vi "Init.vi"(0 "object in":refnum<class "Scripting.lvclass">, 1 "FindAnyOfTheseClassTypes":string[](array[string]), 2 "StopWhenAnyOfTheseClassTypesAreReached":string[](array[string]), 3 "KeepObjectsOpen(True)":bool=TRUE, 4 "DeleteWires(False)":bool, 5 "error in (no error)":errorcluster) -> (14 "object out":refnum<class "Scripting.lvclass">, 19 "error out":errorcluster)   [LabVIEW 2020, in "Scripting.lvclass"]
uses:
  <resource>/Framework/Providers/Open_GDS/ClassProviders/Common/ScriptingFunctions/Scripting.lvclass
  <resource>/Framework/Providers/Open_GDS/ClassProviders/Common/ScriptingFunctions/Scripting.lvclass/Scripting.ctl
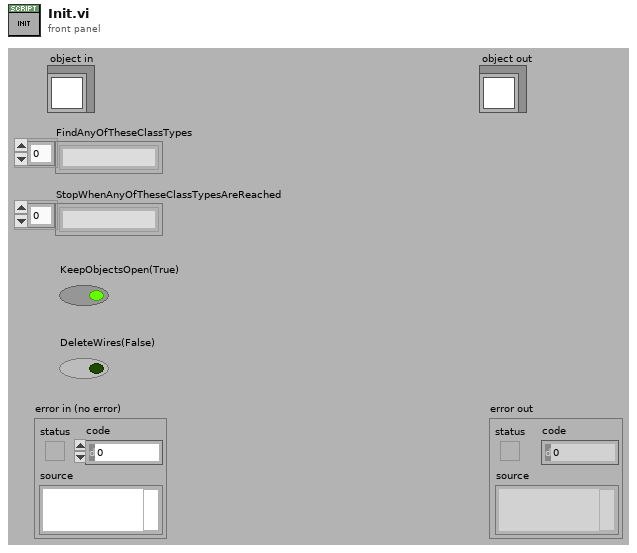
[diagram p1: front panel]
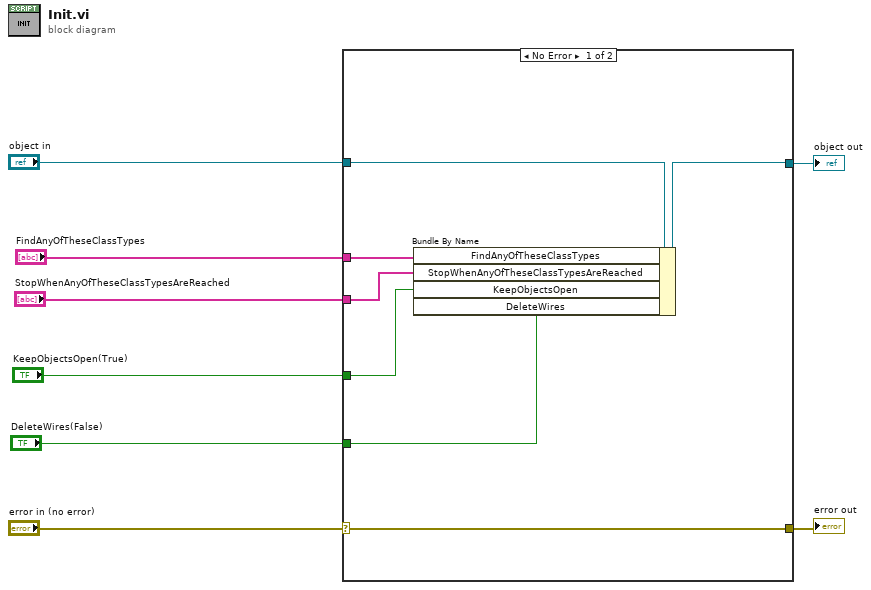
[diagram p0: block diagram]
diagram:
  n1 = case shown="No Error" "error in (no error)" {
    selector: "error in (no error)" -> [w15 w17]
    tunnel: [w15 w17] -> w7
    tunnel: [w13 w16] -> w5
    tunnel: "object in" -> [w14 w16]
    tunnel: "FindAnyOfTheseClassTypes" -> [w12 _]
    tunnel: "StopWhenAnyOfTheseClassTypesAreReached" -> [w11 _]
    tunnel: "KeepObjectsOpen(True)" -> [w10 _]
    tunnel: "DeleteWires(False)" -> [w9 _]
    frame No Error {
      n2 = Bundle By Name(cluster=w14, "FindAnyOfTheseClassTypes"=w12, "StopWhenAnyOfTheseClassTypesAreReached"=w11, "KeepObjectsOpen"=w10, "DeleteWires"=w9) -> (w13:refnum<class "Scripting.lvclass">)
    }
    frame Error {
    }
  }
  "error out" <- w7
  "object out" <- w5
